vi "status.vi"() -> ()   [LabVIEW 2023]
panel:
  out "Auto Scar Check":cluster{"String 2":string}
  # "Camera Initialization in Progress"
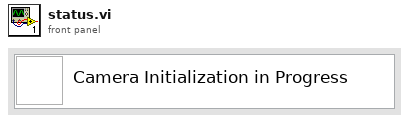
[diagram p1: front panel]
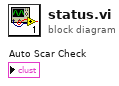
[diagram p0: block diagram]
diagram:
